vi "rqp_Set Place.vi"(4 "Show in Debugger?":bool=TRUE, 6 "Message Priority":T1=enum."Normal", 7 "Caller in":refnum<class "Worker.lvclass">, 8 "error in":errorcluster, 10 "Data in":T2, 11 "Place Temperature in":refnum<class "Place Temperature.lvclass">) -> (0 "error out":errorcluster, 3 "dup Place Temperature out":refnum<class "Place Temperature.lvclass">, 5 "dup Caller out":refnum<class "Worker.lvclass">)   [LabVIEW 2024, in "Place Temperature.lvclass"]
doc: "This VI sends a <b>Public API Request</b> message to an MHL case of the Worker that owns this VI.\n---\nWorkers Public API Request Case"
uses:
  Place Temperature.lvclass
  C:/Program Files (x86)/National Instruments/LabVIEW 2024/vi.lib/addons/_Workers/Library/Classes/Worker/Worker.lvclass
  <vilib>/addons/_Workers/Library/Classes/Worker/Worker.lvclass
  rqp_Set Place.ctl
  <vilib>/addons/_Workers/Library/Classes/Message/Priority.ctl
  <vilib>/addons/_Workers/Library/Case Label.ctl
  <vilib>/addons/_Workers/Library/Classes/Message Queue/Message Queue.lvclass
  Place Temperature.lvclass/Place Temperature.ctl
  <vilib>/addons/_Workers/Library/Workers.lvlib
  <vilib>/addons/_Workers/Library/Classes/Message/Message.lvclass
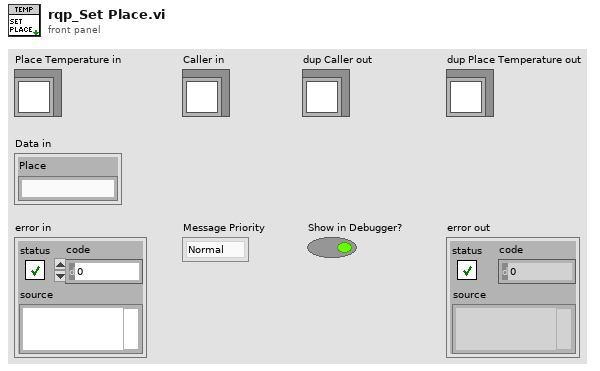
[diagram p1: front panel]
types:
  T1 = typedef "Workers.lvlib/Message.lvclass/Priority.ctl" = enum16{"Low", "Normal", "High"}
  T2 = typedef "Place Temperature.lvclass/rqp_Set Place.ctl" = cluster{"Place":string}
  T3 = typedef "Workers.lvlib/Case Label.ctl" = string
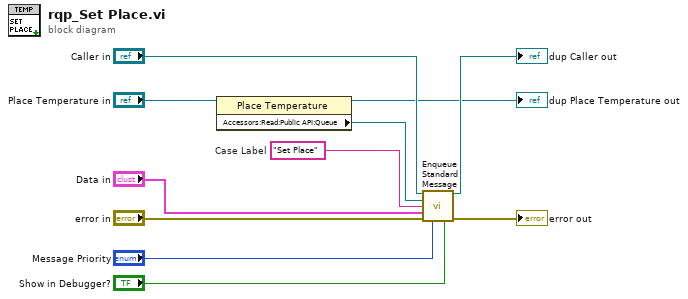
[diagram p0: block diagram]
diagram:
  w1 = T3 "Set Place"  # Case Label
  n1 = property class="Place Temperature"(reference="Place Temperature in") -> (reference out=→"dup Place Temperature out":refnum<class "Place Temperature.lvclass">, "Accessors:Read:Public API:Queue"=w2:refnum<class "Message Queue.lvclass">)  [unwired: 1 in, 1 out]
  n2 = call-dynamic "Enqueue Standard Message.vi"("Worker"="Caller in", "Message Queue"=w2, "Case Label"=w1, "Data"="Data in", "error in (no error)"="error in", "Priority (Normal)"="Message Priority", "Send Message to Debugger? (T)"="Show in Debugger?") -> ("dup Worker out"=→"dup Caller out":refnum<class "Worker.lvclass">, "error out"=→"error out":errorcluster)  [unwired: 7 in]
